vi "Read Content Bounds.vi"(8 "error in (no error)":errorcluster, 11 "SceneGraphDisplay.lvclass in":refnum<class "SceneGraphDisplay.lvclass">) -> (0 "error out":errorcluster, 2 "ContentBounds":T1, 3 "SceneGraphDisplay.lvclass out":refnum<class "SceneGraphDisplay.lvclass">)   [LabVIEW 2015, in "SceneGraphDisplay.lvclass"]
uses:
  SceneGraphDisplay.lvclass
  <vilib>/Utility/miscctls.llb/LVBoundsTypeDef.ctl
  SceneGraphDisplay.lvclass/SceneGraphDisplay.ctl
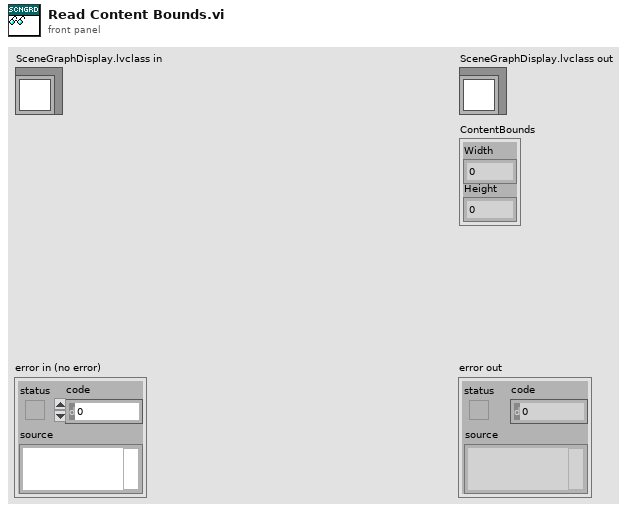
[diagram p1: front panel]
types:
  T1 = typedef "LVBoundsTypeDef.ctl" = cluster{"Width":u32, "Height":u32}
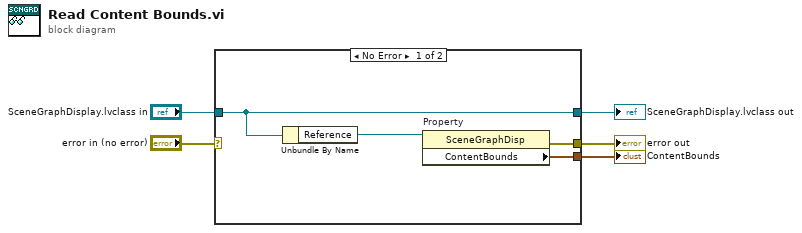
[diagram p0: block diagram]
diagram:
  n1 = case shown="No Error" "error in (no error)" {
    selector: "error in (no error)" -> [_ w11]
    tunnel: [w8 w11] -> w4
    tunnel: [w7 w10] -> w2
    tunnel: "SceneGraphDisplay.lvclass in" -> [w7 w10]
    tunnel: [w9 _] -> w1
    frame No Error {
      n2 = Unbundle By Name(w7) -> ("Reference"=w6:refnum<vi>)
      n3 = property on="Property" class="SceneGraphDisp"(reference=w6) -> (error out=w8:errorcluster, "ContentBounds"=w9:T1)  [unwired: 1 in, 1 out]
    }
    frame Error {
    }
  }
  "error out" <- w4
  "SceneGraphDisplay.lvclass out" <- w2
  "ContentBounds" <- w1
